vi "create_filename.vi"(11 "series_class in":refnum<class "series_class.lvclass">) -> (2 "json filename":string, 3 "series_class out":refnum<class "series_class.lvclass">)   [LabVIEW 2024, in "series_class.lvclass"]
uses:
  series_class.lvclass
  series_class.lvclass/series_class.ctl
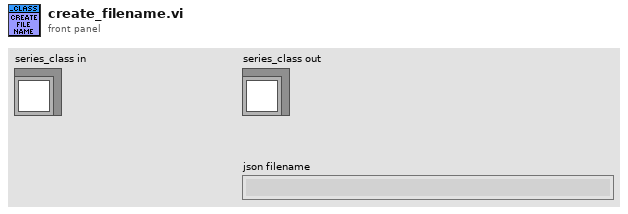
[diagram p1: front panel]
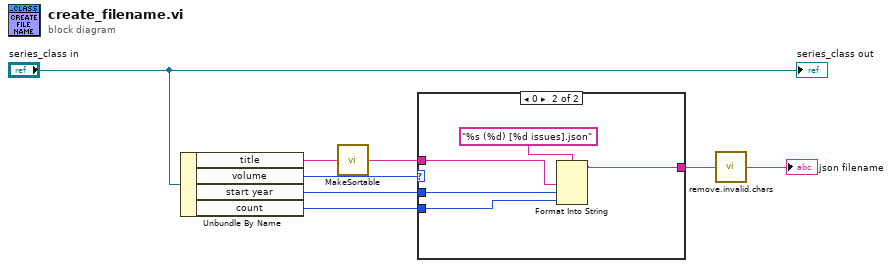
[diagram p0: block diagram]
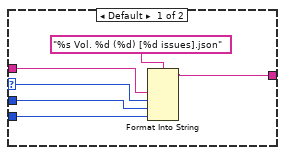
[diagram p2: hidden frame]
diagram:
  n1 = Unbundle By Name("series_class in") -> ("title"=w7:string, "volume"=w3:i32, "start year"=w5:i32, "count"=w4:i32)
  n2 = call "MakeSortable.vi"("string in"=w7) -> ("string out"=w6:string)
  n3 = case shown="0" w3 {
    selector: w3 -> [w9 _]
    tunnel: [w14 w19] -> w2
    tunnel: w6 -> [w12 w17]
    tunnel: w5 -> [w11 w16]
    tunnel: w4 -> [w10 w15]
    frame Default {
      n4 = Format Into String(format string="%s Vol. %d (%d) [%d issues].json", w12, w9, w11, w10) -> (resulting string=w14:string)  [unwired: 2 in, 1 out]
    }
    frame 0 {
      n5 = Format Into String(format string="%s (%d) [%d issues].json", w17, w16, w15) -> (resulting string=w19:string)  [unwired: 2 in, 1 out]
    }
  }
  n6 = call "remove.invalid.chars.vi"("string in"=w2) -> ("string out"=→"json filename":string)
  "series_class out" <- "series_class in"
